vi "add prefix suffix test.vi"() -> (0 "error out":errorcluster, 3 "Tag location the same?":bool)   [LabVIEW 2015, in "E2E Tag Exchange tests.lvlib"]
uses:
  E2E Tag Exchange tests.lvlib
  <vilib>/NI/Module Execution Interface/Engine Configuration/engine configuration.lvclass
  <vilib>/NI/Tag Bus Module Framework/channel/channel classification.ctl
  <vilib>/NI/Configuration Framework/serializable configuration/NISE_CEF_serializable configuration.lvclass/NISE_CEF_serializable configuration.ctl
  module/configuration/E2E Tag Exchange configuration.lvclass/E2E Tag Exchange configuration.ctl
  <vilib>/NI/Tag Bus/tag/tag descriptor.lvclass/tag descriptor.ctl
  <vilib>/Utility/LVClass/Get LV Class Name.vi
  <vilib>/NI/Configuration Framework/error generator/NISE_error generator.vi
  module/configuration/E2E Tag Exchange configuration.lvclass
  <vilib>/NI/Configuration Framework/serializable configuration/NISE_CEF_serializable configuration.lvclass
  editor node/E2E Tag Exchange editor node.lvclass
  <vilib>/NI/Tag Bus Module Framework/channel/TBM channel.lvclass
  <vilib>/NI/Tag Bus/dictionary/data dictionary.lvclass
  <vilib>/NI/Tag Bus/tag/tag descriptor.lvclass
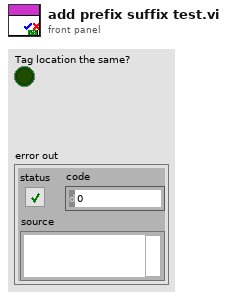
[diagram p1: front panel]
types:
  T1 = typedef "TBM channel.lvclass/channel classification.ctl" = enum16{"input data", "output data", "processing parameter", "processing result"}
  T2 = typedef "TBM channel.lvclass/data tables.ctl" = cluster{"input data":T3, "processing parameter":T3, "processing result":T3, "output data":T3}
  T3 = typedef "tag bus.lvlib/dictionary table pair.ctl" = cluster{"data dictionary":refnum<class "data dictionary.lvclass">, "data table":T4}
  T4 = typedef "tag bus.lvlib/data table.lvlib/data table.ctl" = cluster{"Double":dbl[], "Single":sgl[], "I64":i64[], "I32":i32[], "I16":i16[], "I8":i8[], "U64":u64[], "U32":u32[], "U16":u16[], "U8":u8[], "Boolean":bool[], "String":string[], "Array of Double":cluster{"DBL Array":dbl[]}[], "Array of Single":cluster{"SGL Array":sgl[]}[], "Array of I64":cluster{"I64 Array":i64[]}[], "Array of I32":cluster{"I32 Array":i32[]}[], "Array of I16":cluster{"I16 Array":i16[]}[], "Array of I8":cluster{"I8 Array":i8[]}[], "Array of U64":cluster{"U64 Array":u64[]}[], "Array of U32":cluster{"U32 Array":u32[]}[], "Array of U16":cluster{"U16 Array":u16[]}[], "Array of U8":cluster{"U8 Array":u8[]}[], "Array of Boolean":cluster{"Boolean Array":bool[]}[], "Array of String":cluster{"String Array":string[]}[]}
  T5 = typedef "tag bus.lvlib/tag descriptor.lvclass/Data Type.ctl" = enum16{"Double", "Single", "I64", "I32", "I16", "I8", "U64", "U32", "U16", "U8", "Boolean", "String", "Array of Double", "Array of Single", "Array of I64", "Array of I32", "Array of I16", "Array of I8", "Array of U64", "Array of U32", "Array of U16", "Array of U8", "Array of Boolean", "Array of String"}
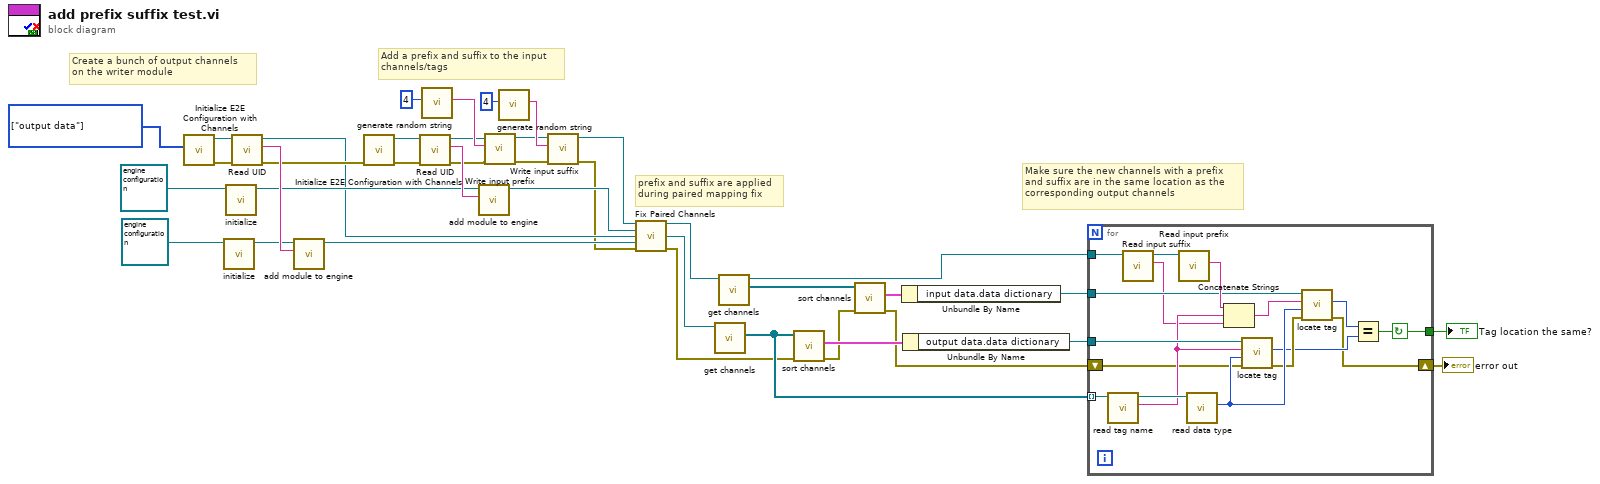
[diagram p0: block diagram]
diagram:
  w22 = T1[] [enum."output data"] items=["input data", "output data", "processing parameter", "processing result"] ("Supported Channel Classifications (All)")
  # "Make sure the new channels with a prefix\nand suffix are in the same location as the \ncorresponding output channels"
  # "prefix and suffix are applied\nduring paired mapping fix"
  # "Add a prefix and suffix to the input\nchannels/tags"
  # "Create a bunch of output channels\non the writer module"
  n1 = call "Initialize E2E Configuration with Channels.vi"("Supported Channel Classifications (All)"=w22) -> ("error out"=w35:errorcluster, "Initialized E2E configuration"=w34:refnum<class "E2E Tag Exchange configuration.lvclass">)  [unwired: 8 in, 1 out]
  n2 = call <vilib>:"initialize.vi"("configuration in"=refnum<class "engine configuration.lvclass"> refnum ("engine configuration")) -> ("configuration out"=w31:refnum<class "engine configuration.lvclass">)  [unwired: 8 in, 2 out]
  n3 = call <vilib>:"initialize.vi"("configuration in"=refnum<class "engine configuration.lvclass"> refnum ("engine configuration")) -> ("configuration out"=w30:refnum<class "engine configuration.lvclass">)  [unwired: 8 in, 2 out]
  n4 = call <vilib>:"Read UID.vi"("error in"=w35, "configuration in"=w34) -> ("error out"=w9:errorcluster, "instance id"=w39:string, "configuration out"=w8:refnum<class "E2E Tag Exchange configuration.lvclass">)  [unwired: 7 in]
  n5 = call-dynamic "add module to engine.vi"("module ID"=w39, "engine configuration in"=w31) -> ("engine configuration out"=w32:refnum<class "engine configuration.lvclass">)  [unwired: 8 in, 1 out]
  n6 = call "Initialize E2E Configuration with Channels.vi"("error in"=w9) -> ("error out"=w37:errorcluster, "Initialized E2E configuration"=w36:refnum<class "E2E Tag Exchange configuration.lvclass">)  [unwired: 8 in, 1 out]
  n7 = call <vilib>:"Read UID.vi"("error in"=w37, "configuration in"=w36) -> ("error out"=w6:errorcluster, "instance id"=w38:string, "configuration out"=w7:refnum<class "E2E Tag Exchange configuration.lvclass">)  [unwired: 7 in]
  n8 = call "generate random string.vi"("Number of Characters"=4) -> ("string"=w27:string)  [unwired: 10 in]
  n9 = call-dynamic "add module to engine.vi"("module ID"=w38, "engine configuration in"=w30) -> ("engine configuration out"=w33:refnum<class "engine configuration.lvclass">)  [unwired: 8 in, 1 out]
  n10 = call "Write input prefix.vi"("error in (no error)"=w6, "input prefix"=w27, "E2E Tag Exchange configuration in"=w7) -> ("error out"=w4:errorcluster, "E2E Tag Exchange configuration out"=w5:refnum<class "E2E Tag Exchange configuration.lvclass">)  [unwired: 7 in]
  n11 = call "generate random string.vi"("Number of Characters"=4) -> ("string"=w26:string)  [unwired: 10 in]
  n12 = call "Write input suffix.vi"("error in (no error)"=w4, "paired output suffix"=w26, "E2E Tag Exchange configuration in"=w5) -> ("error out"=w3:errorcluster, "E2E Tag Exchange configuration out"=w2:refnum<class "E2E Tag Exchange configuration.lvclass">)  [unwired: 7 in]
  n13 = call "Fix Paired Channels.vi"("Paired E2E configuration in"=w2, "Paired engine configuration in"=w33, "E2E configuration in"=w8, "engine configuration in"=w32, "error in (no error)"=w3) -> ("Paired E2E configuration out"=w21:refnum<class "E2E Tag Exchange configuration.lvclass">, "E2E configuration out"=w1:refnum<class "E2E Tag Exchange configuration.lvclass">, "error out"=w13:errorcluster)  [unwired: 6 in, 2 out]
  n14 = call-dynamic "get channels.vi"("E2E configuration in"=w1) -> ("channels"=w18:refnum<class "TBM channel.lvclass">[])  [unwired: 9 in, 1 out]
  n15 = call-dynamic "get channels.vi"("E2E configuration in"=w21) -> ("channels"=w20:refnum<class "TBM channel.lvclass">[], "E2E configuration out"=w15:refnum<class "E2E Tag Exchange configuration.lvclass">)  [unwired: 9 in]
  n16 = call <vilib>:"sort channels.vi"("error in"=w13, "channels in"=w18) -> ("error out"=w12:errorcluster, "data allocations"=w19:T2)  [unwired: 7 in, 1 out]
  n17 = call <vilib>:"sort channels.vi"("error in"=w12, "channels in"=w20) -> ("error out"=w11:errorcluster, "data allocations"=w23:T2)  [unwired: 7 in, 1 out]
  n18 = Unbundle By Name(w23) -> ("input data.data dictionary"=w16:refnum<class "data dictionary.lvclass">)
  n19 = Unbundle By Name(w19) -> ("output data.data dictionary"=w17:refnum<class "data dictionary.lvclass">)
  n20 = for {
    tunnel: w18 -> [w56] mode=indexing
    tunnel: w15 -> [w53]
    tunnel: w17 -> [w55]
    tunnel: w16 -> [w49]
    tunnel: [w42] -> w14
    shift-right: [w41] -> w10
    shift-left: w11 -> [w43]
    stop <- w42 continue-if-true
    n21 = call <vilib>:"read tag name.vi"("system tag in"=w56) -> ("name"=w52:string, "system tag out"=w54:refnum<class "TBM channel.lvclass">)  [unwired: 8 in, 1 out]
    n22 = call "Read input suffix.vi"("E2E Tag Exchange configuration in"=w53) -> ("input suffix"=w40:string, "E2E Tag Exchange configuration out"=w51:refnum<class "E2E Tag Exchange configuration.lvclass">)  [unwired: 8 in, 1 out]
    n23 = call "Read input prefix.vi"("E2E Tag Exchange configuration in"=w51) -> ("input prefix"=w50:string)  [unwired: 8 in, 2 out]
    n24 = call <vilib>:"read data type.vi"("system tag in"=w54) -> ("data type"=w47:T5)  [unwired: 8 in, 2 out]
    n25 = Concatenate Strings(w50, w52, w40) -> (w48:string)
    n26 = call <vilib>:"locate tag.vi"("error in"=w43, "data type"=w47, "name"=w52, "data dictionary in"=w55) -> ("error out"=w46:errorcluster, "index"=w44:i32)  [unwired: 5 in, 1 out]
    n27 = call <vilib>:"locate tag.vi"("error in"=w46, "data type"=w47, "name"=w48, "data dictionary in"=w49) -> ("error out"=w41:errorcluster, "index"=w45:i32)  [unwired: 5 in, 1 out]
    n28 = Equal?(x=w45, y=w44) -> (x = y?=w42:bool)
  }
  "Tag location the same?" <- w14
  "error out" <- w10
